vi "Sync Test.vi"() -> ()   [LabVIEW 2010]
uses:
  <vilib>/Platform/TimedLoop/XDataNode/XDataNode.xnode
  <vilib>/Platform/TimedLoop/XDataNode/timing_clust.ctl
  <vilib>/Platform/TimedLoop/XDataNode/nitl_modes.ctl
  <vilib>/Platform/TimedLoop/XDataNode/wakeup.ctl
  <vilib>/DAQmx/write.llb/DAQmx Write (Analog DBL 1Chan 1Samp).vi
  <vilib>/DAQmx/create/channels.llb/DAQmx Create Channel (AO-Voltage-Basic).vi
  <vilib>/DAQmx/configure/timing.llb/DAQmx Timing (Sample Clock).vi
  <vilib>/xnet/xnet.llb/XNET Create Session (Signal Input Single-point).vi
  <vilib>/xnet/xnet.llb/XNET Create Session (Signal Output Single-point).vi
  <vilib>/xnet/xnet.llb/XNET Create Timing Source (FlexRay Cycle).vi
  <vilib>/xnet/xnet.llb/XNET Read (State FlexRay Cycle Macrotick).vi
  <vilib>/daqmx/miscellaneous.llb/DAQmx Fill In Error Info.vi
  <vilib>/Platform/TimedLoop/XDataNode/XDNodeRunTimeDep.lvlib
panel:
  in  "Select":bool caption="Each VI running needs this switch set different!"
  out "dt":u32
  out "error out":errorcluster
  in  "stop":bool
  # "VI1: set high\nVI2: set low"
  # "uS"
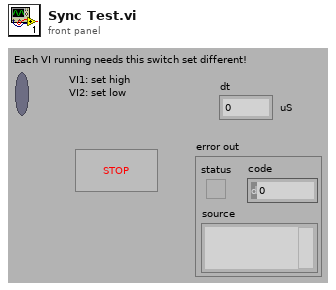
[diagram p1: front panel]
types:
  T1 = typedef "XDNodeRunTimeDep.lvlib/timing_clust.ctl" = cluster{"Expected End [f-1]":u64, "Actual End [f-1]":u64, "Finished Late? [f-1]":bool, "Expected End [i-1]":u64, "Actual End [i-1]":u64, "Finished Late? [i-1]":bool, "Expected Start [i]":u64, "Actual Start [i]":u64, "Expected Start [f]":u64, "Actual Start [f]":u64, "Source Name":string, "Structure Name":string, "Period":i64, "Deadline":i64, "Offset":i64, "Start":i64, "Priority":i32, "Timeout":i32, "Mode":T2, "Wakeup Reason":T3, "Error":errorcluster, "Source Type":string, "Secondary Source Type":string, "Global End Time":u64, "Global Start Time":u64, "Frame Duration":u64, "Iteration Duration":u64, "Assigned CPU":i32, "I/O Scan Engine Mode":u32}
  T2 = typedef "XDNodeRunTimeDep.lvlib/nitl_modes.ctl" = enum32{"No Change", "Process missed periods, maintain original phase", "Discard missed periods, maintain original phase", "Process missed periods, ignore original phase", "Discard missed periods, ignore original phase"}
  T3 = typedef "XDNodeRunTimeDep.lvlib/wakeup.ctl" = enum32{"Normal", "Aborted", "Asynchronous wakeup", "Timing source error", "Timed loop error", "Timeout"}
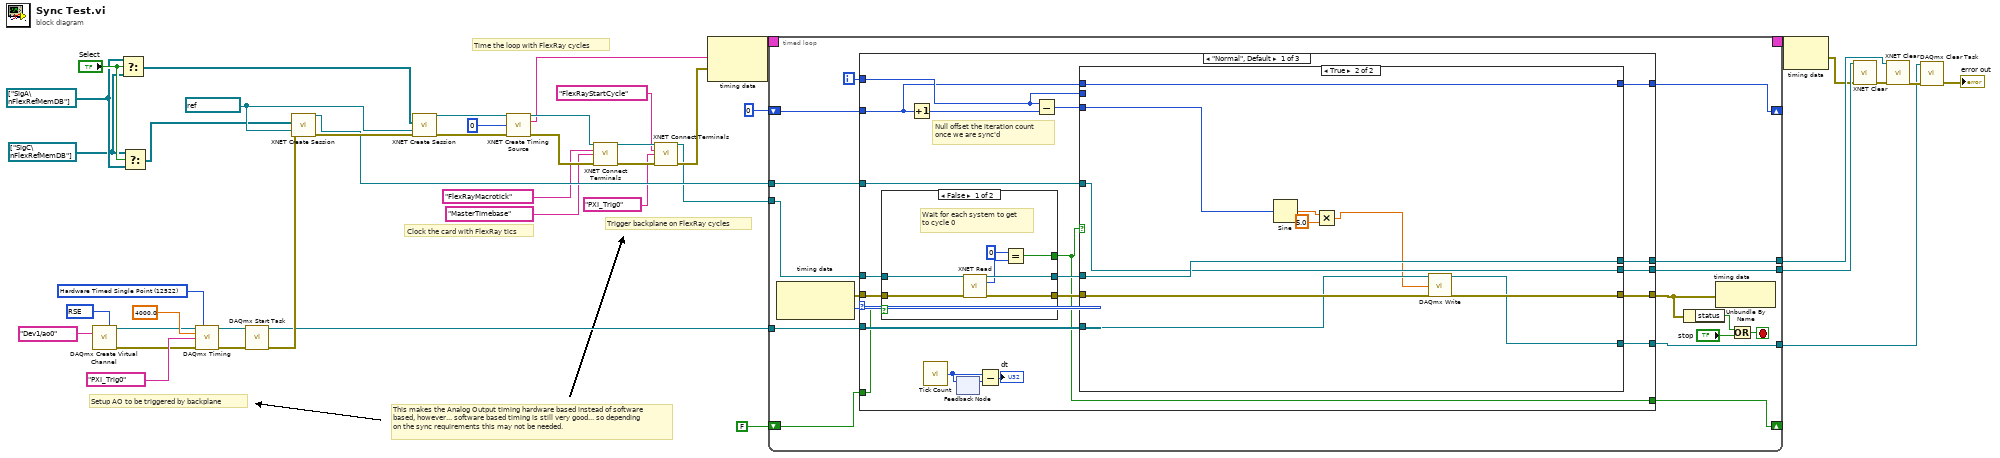
[diagram p0: block diagram]
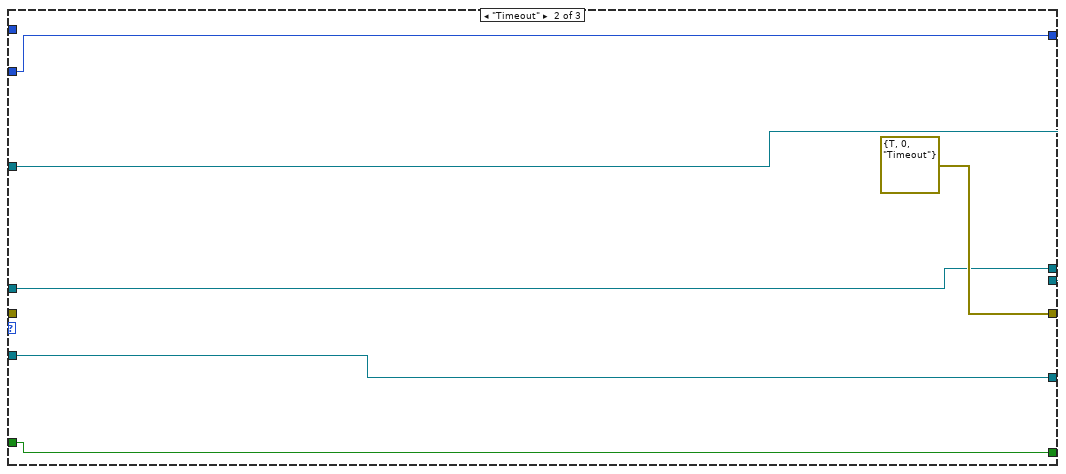
[diagram p4: hidden frame]
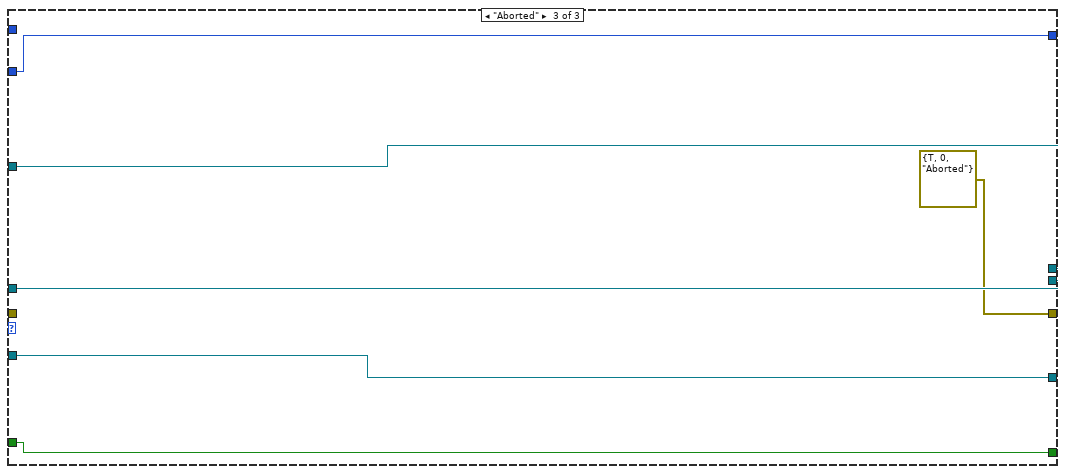
[diagram p5: hidden frame]
diagram:
  w9 = 12522 items=["Finite Samples"=10178, "Continuous Samples"=10123, "Hardware Timed Single Point"=12522] ("sample mode")
  w18 = refnum<k21>[] ["SigC\nFlexRefMemDB"] ("signal list")
  w19 = refnum<k21>[] ["SigA\nFlexRefMemDB"] ("signal list")
  w32 = 10083 items=["Default"=-1, "RSE"=10083, "Differential"=10106, "Pseudodifferential"=12529] ("output terminal configuration")
  w40 = refnum<k21> "FlexRay1" ("interface")
  # "This makes the Analog Output timing hardware based instead of software based, however... software based timing is still very good... so depending on the sync requirements this may not be needed."
  # "Setup AO to be triggered by backplane"
  # "Trigger backplane on FlexRay cycles"
  # "Clock the card with FlexRay tics"
  # "Time the loop with FlexRay cycles"
  n1 = call-poly <vilib>:"DAQmx Create Virtual Channel.vi"("output terminal configuration"=w32, "physical channels"=tag "Dev1/ao0") -> ("task out"=w5:refnum<k21>, "error out"=w6:errorcluster)  [unwired: 12 in]
  n2 = Select(t=w19, s="Select", f=w18) -> (s? t:f=w16:refnum<k21>[])
  n3 = Select(t=w18, s="Select", f=w19) -> (s? t:f=w17:refnum<k21>[])
  n4 = call-poly <vilib>:"DAQmx Timing.vi"("task/channels in"=w5, "sample mode"=w9, "rate"=4000.0, "source"=tag "PXI_Trig0", "error in"=w6) -> ("task out"=w3:refnum<k21>, "error out"=w4:errorcluster)  [unwired: 9 in]
  n5 = call <vilib>:"DAQmx Start Task.vi"("task/channels in"=w3, "error in"=w4) -> ("task out"=w1:refnum<k21>, "error out"=w2:errorcluster)  [unwired: 12 in]
  n6 = call-poly <vilib>:"XNET Create Session.vi"("signal list"=w17, "interface"=w40, "error in (no error)"=w2) -> ("session out"=w33:refnum<k21>, "error out"=w39:errorcluster)  [unwired: 11 in]
  n7 = call-poly <vilib>:"XNET Create Session.vi"("signal list"=w16, "interface"=w40, "error in (no error)"=w39) -> ("session out"=w35:refnum<k21>, "error out"=w36:errorcluster)  [unwired: 11 in]
  n8 = call-poly <vilib>:"XNET Create Timing Source.vi"("session in"=w35, "macrotick offset"=u32 0, "error in (no error)"=w36) -> ("session out"=w27:refnum<k21>, "timing source out"=w22:string, "error out"=w28:errorcluster)  [unwired: 10 in]
  n9 = call <vilib>:"XNET Connect Terminals.vi"("session in"=w27, "source terminal"=tag "FlexRayMacrotick" ("XNET Terminal"), "destination terminal"=tag "MasterTimebase" ("XNET Terminal"), "error in (no error)"=w28) -> ("session out"=w14:refnum<k21>, "error out"=w15:errorcluster)  [unwired: 10 in]
  n10 = call <vilib>:"XNET Connect Terminals.vi"("session in"=w14, "source terminal"=tag "FlexRayStartCycle", "destination terminal"=tag "PXI_Trig0" ("source terminal"), "error in (no error)"=w15) -> ("session out"=w12:refnum<k21>, "error out"=w13:errorcluster)  [unwired: 10 in]
  n11 = node-c288(w22, w13) -> (w44:T1)
  n12 = timed-loop {
    timing: w44 -> [_]
    timing-out: [_] -> w43
    tunnel: w12 -> [w51]
    tunnel: [w61] -> w42
    tunnel: w33 -> [w56]
    tunnel: [w59] -> w41
    tunnel: w1 -> [w58]
    tunnel: [w57] -> w30
    shift-right: [w45] -> _
    shift-left: 0 -> [w47]
    shift-right: [w48] -> _
    shift-left: FALSE -> [w49]
    i -> [w46]
    stop <- w52 stop-if-true
    n13 = node-c288() -> (w50:errorcluster, w60:T3)  [unwired: 1 in]
    n14 = case shown="\"Normal\", Default" w60 {
      tunnel: w50 -> [w75 _ _]
      tunnel: w51 -> [w74 w111 w119]
      tunnel: [w81 w111 w119] -> w61
      tunnel: [w78 errorcluster {"status"=TRUE, "code"=0, "source"="Timeout"} ("Error") errorcluster {"status"=TRUE, "code"=0, "source"="Aborted"} ("Error")] -> w53
      tunnel: w56 -> [w80 w112 w117]
      tunnel: [w79 w112 w117] -> w59
      tunnel: w58 -> [w77 w110 w116]
      tunnel: [w76 w110 w116] -> w57
      tunnel: w49 -> [w71 w109 w115]
      tunnel: [w70 w109 w115] -> w48
      tunnel: w47 -> [w63 w108 w114]
      tunnel: w46 -> [w64 _ _]
      tunnel: [w62 w108 w114] -> w45
      frame "Normal", Default {
        # "Null offset the iteration count\nonce we are sync'd"
        n15 = case shown="False" w71 {
          selector: w71 -> [_ w89]
          tunnel: w75 -> [w88 w90]
          tunnel: [w87 w90] -> w72
          tunnel: [w86 w91] -> w73
          tunnel: w74 -> [w85 w91]
          tunnel: [w83 w89] -> w70
          frame False {
            # "Wait for each system to get\nto cycle 0"
            n16 = call-poly <vilib>:"XNET Read.vi"("session in"=w85, "error in (no error)"=w88) -> ("session out"=w86:refnum<k21>, "cycle"=w84:u8, "error out"=w87:errorcluster)  [unwired: 10 in, 1 out]
            n17 = Equal?(x=u8 0, y=w84) -> (x = y?=w83:bool)
          }
          frame True {
          }
        }
        n18 = Increment(x=w63) -> (x+1=w66:i32)
        n19 = call "Tick Count"() -> ("Tick Count(uSec)"=w68:u32)
        n20 = feedback #1() -> (w69:u32)  [unwired: 1 in]
        n21 = feedback-in #1(w68) -> ()
        n22 = Subtract(x=w68, y=w69) -> (x-y=→"dt":u32)
        n23 = Subtract(x=w64, y=w66) -> (x-y=w65:i32)
        n24 = case shown="True" w70 {
          tunnel: w65 -> [_ w100]
          tunnel: w73 -> [w94 w106]
          tunnel: w72 -> [w93 w107]
          tunnel: [w95 w106] -> w81
          tunnel: w80 -> [w95 w101]
          tunnel: [w94 w101] -> w79
          tunnel: [w93 w105] -> w78
          tunnel: w77 -> [w92 w104]
          tunnel: [w92 w103] -> w76
          tunnel: w64 -> [w96 _]
          tunnel: w63 -> [_ w102]
          tunnel: [w96 w102] -> w62
          frame False {
            # "Still waiting for cycles on each target to sync to 0."
          }
          frame True {
            n25 = Sine(x=w100) -> (sin(x)=w99:dbl)
            n26 = Multiply(x=w99, y=5.0) -> (x*y=w97:dbl)
            n27 = call-poly <vilib>:"DAQmx Write.vi"("task/channels in"=w104, "data"=w97, "error in"=w107) -> ("task out"=w103:refnum<k21>, "error out"=w105:errorcluster)  [unwired: 10 in, 1 out]
          }
        }
      }
      frame "Timeout" {
      }
      frame "Aborted" {
      }
    }
    n28 = Unbundle By Name(w53) -> ("status"=w54:bool)
    n29 = node-c288(w53) -> ()  [unwired: 1 out]
    n30 = Or(x=w54, y="stop") -> (x .or. y?=w52:bool)
  }
  n31 = node-c288(w43) -> (w38:errorcluster)
  n32 = call <vilib>:"XNET Clear.vi"("session in"=w41, "error in (no error)"=w38) -> ("error out"=w37:errorcluster)  [unwired: 13 in]
  n33 = call <vilib>:"XNET Clear.vi"("session in"=w42, "error in (no error)"=w37) -> ("error out"=w31:errorcluster)  [unwired: 13 in]
  n34 = call <vilib>:"DAQmx Clear Task.vi"("task in"=w30, "error in"=w31) -> ("error out"=→"error out":errorcluster)  [unwired: 13 in]
